vi "mask_circular.vi"(8 "clu_mask_cor":T1, 11 "image in":T2) -> (3 "masekd image out":T2)   [LabVIEW 2011]
uses:
  <vilib>/vision/Image Controls.llb/IMAQ Image.ctl
  <vilib>/vision/NI_Vision_Development_Module.lvlib
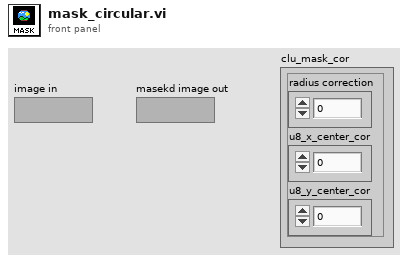
[diagram p1: front panel]
types:
  T1 = cluster{"radius correction":i16, "u8_x_center_cor":i16, "u8_y_center_cor":i16}
  T2 = typedef "IMAQ Image.ctl" = refnum<image>
  T3 = typedef "IMAQ Circle" = cluster{"Center X":i32, "Center Y":i32, "Inner Radius":i32, "Outer Radius":i32, "Start Angle":dbl, "End Angle":dbl}
  T4 = typedef "Image Type" = u32
  T5 = typedef "ROI Descriptor" = cluster{"Global Rectangle":i32[], "Contours":cluster{"ID":enum32{"External", "Internal"}, "Type":u32, "Coordinates":i32[]}[]}
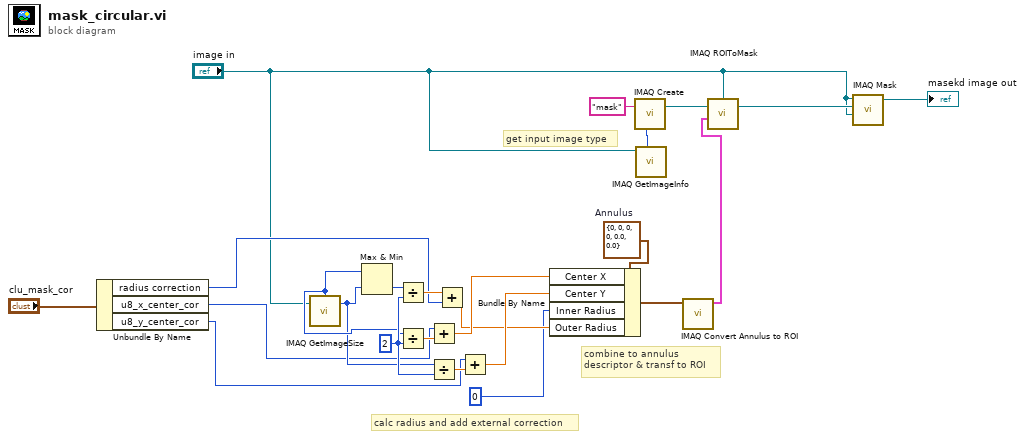
[diagram p0: block diagram]
diagram:
  w17 = T3 {"Center X"=0, "Center Y"=0, "Inner Radius"=0, "Outer Radius"=0, "Start Angle"=0.0, "End Angle"=0.0}  # Annulus
  w20 = 2 ("y")
  # "get input image type"
  # "combine to annulus\ndescriptor & transf to ROI"
  # "calc radius and add external correction"
  n1 = Unbundle By Name("clu_mask_cor") -> ("radius correction"=w7:i16, "u8_x_center_cor"=w6:i16, "u8_y_center_cor"=w5:i16)
  n2 = call "IMAQ GetImageSize"("Image"="image in") -> ("Y Resolution"=w15:i32, "X Resolution"=w16:i32)  [unwired: 3 in, 1 out]
  n3 = Max & Min(x=w16, y=w15) -> (min(x,y)=w19:i32)  [unwired: 1 out]
  n4 = Divide(x=w19, y=w20) -> (x/y=w21:dbl)
  n5 = Divide(x=w16, y=w20) -> (x/y=w12:dbl)
  n6 = Add(x=w6, y=w12) -> (x+y=w24:dbl)
  n7 = Divide(x=w15, y=w20) -> (x/y=w13:dbl)
  n8 = Add(x=w21, y=w7) -> (x+y=w22:dbl)
  n9 = Add(x=w5, y=w13) -> (x+y=w23:dbl)
  n10 = Bundle By Name(cluster=w17, "Center X"=w24, "Center Y"=w23, "Inner Radius"=0, "Outer Radius"=w22) -> (w18:T3)
  n11 = call "IMAQ GetImageInfo"("Image"="image in") -> ("Image Type"=w1:T4)  [unwired: 3 in, 7 out]
  n12 = call "IMAQ Create"("Image Name"="mask", "Image Type"=w1) -> ("New Image"=w3:T2)  [unwired: 3 in, 1 out]
  n13 = call "IMAQ Convert Annulus to ROI"("Annulus"=w18) -> ("ROI Descriptor"=w11:T5)  [unwired: 8 in, 1 out]
  n14 = call "IMAQ ROIToMask"("ROI Descriptor"=w11, "Image"=w3, "Image Model"="image in") -> ("Image Out"=w9:T2)  [unwired: 2 in, 3 out]
  n15 = call "IMAQ Mask"("Image Dst"="image in", "Image Mask"=w9, "Image Src"="image in") -> ("Image Dst Out"=→"masekd image out":T2)  [unwired: 2 in, 1 out]
